vi "Periodic Tasks.vi"(8 "error in":errorcluster) -> ()   [LabVIEW 2023]
doc: "This VI runs in parallel to other tasks. It can contain as many user-defined periodic loops as you need. These can carry out PID or other sorts of timed response."
uses:
  <vilib>/Rock Robotics/WPI/Utilities/WPI_GetSetVariantRefNum.vi
  Robot Global Data.vi
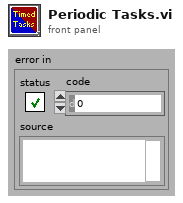
[diagram p1: front panel]
types:
  T1 = typedef "WPI_JoystickDevRef.ctl" = cluster{"Device":T2}
  T2 = typedef "WPI_JoystickDeviceEnum.ctl" = enum16{"USB 0", "USB 1", "USB 2", "USB 3", "USB 4", "USB 5"}
  T3 = typedef "WPI_RobotDriveDevRef.ctl" = cluster{"DevStatus":errorcluster, "Motors[]":T4[], "Square Inputs":bool, "Max Output":dbl}
  T4 = typedef "WPI_MotorControlDeviceRef.ctl" = cluster{"DeviceStatus":errorcluster, "Type":T5, "PWM":cluster{"PWM Channel":T6, "DeadBand":T7}, "CAN":cluster{"Device Number":u8, "SetOutput VI Ref":variant, "GetOutput VI Ref":variant, "Enable VI Ref":variant, "Disable VI Ref":variant, "Data":variant}, "Invert":bool, "DIO PWM":cluster{"PWM \"Enable\" Channel":T6, "DIOChannel":T8, "PWM Rate":dbl}}
  T5 = typedef "WPI_MotorControlType.ctl" = enum16{"PWM", "CAN", "DIO PWM"}
  T6 = typedef "FPGA_DIOPWMChannel.ctl" = enum8{"PWM 0", "PWM 1", "PWM 2", "PWM 3", "PWM 4", "PWM 5", "PWM 6", "PWM 7", "PWM 8", "PWM 9", "PWM MXP 0", "PWM MXP 1", "PWM MXP 2", "PWM MXP 3", "PWM MXP 4", "PWM MXP 5", "PWM MXP 6", "PWM MXP 7", "PWM MXP 8", "PWM MXP 9", "Invalid"}
  T7 = typedef "WPI_PWMDeadband.ctl" = cluster{"Name":string, "maxPositivePwm":i32, "minPositivePwm":i32, "centerPwm":i32, "maxNegativePwm":i32, "minNegativePwm":i32, "angularRange":u16}
  T8 = typedef "FPGA_DIOChannel.ctl" = enum8{"DIO 0", "DIO 1", "DIO 2", "DIO 3", "DIO 4", "DIO 5", "DIO 6", "DIO 7", "DIO 8", "DIO 9", "DIO MXP 0", "DIO MXP 1", "DIO MXP 2", "DIO MXP 3", "DIO MXP 4", "DIO MXP 5", "DIO MXP 6", "DIO MXP 7", "DIO MXP 8", "DIO MXP 9", "DIO MXP 10", "DIO MXP 11", "DIO MXP 12", "DIO MXP 13", "DIO MXP 14", "DIO MXP 15", "SPI Port CS1", "SPI Port CS2", "SPI Port CS3", "SPI Port MISO", "SPI Port MOSI", "Invalid"}
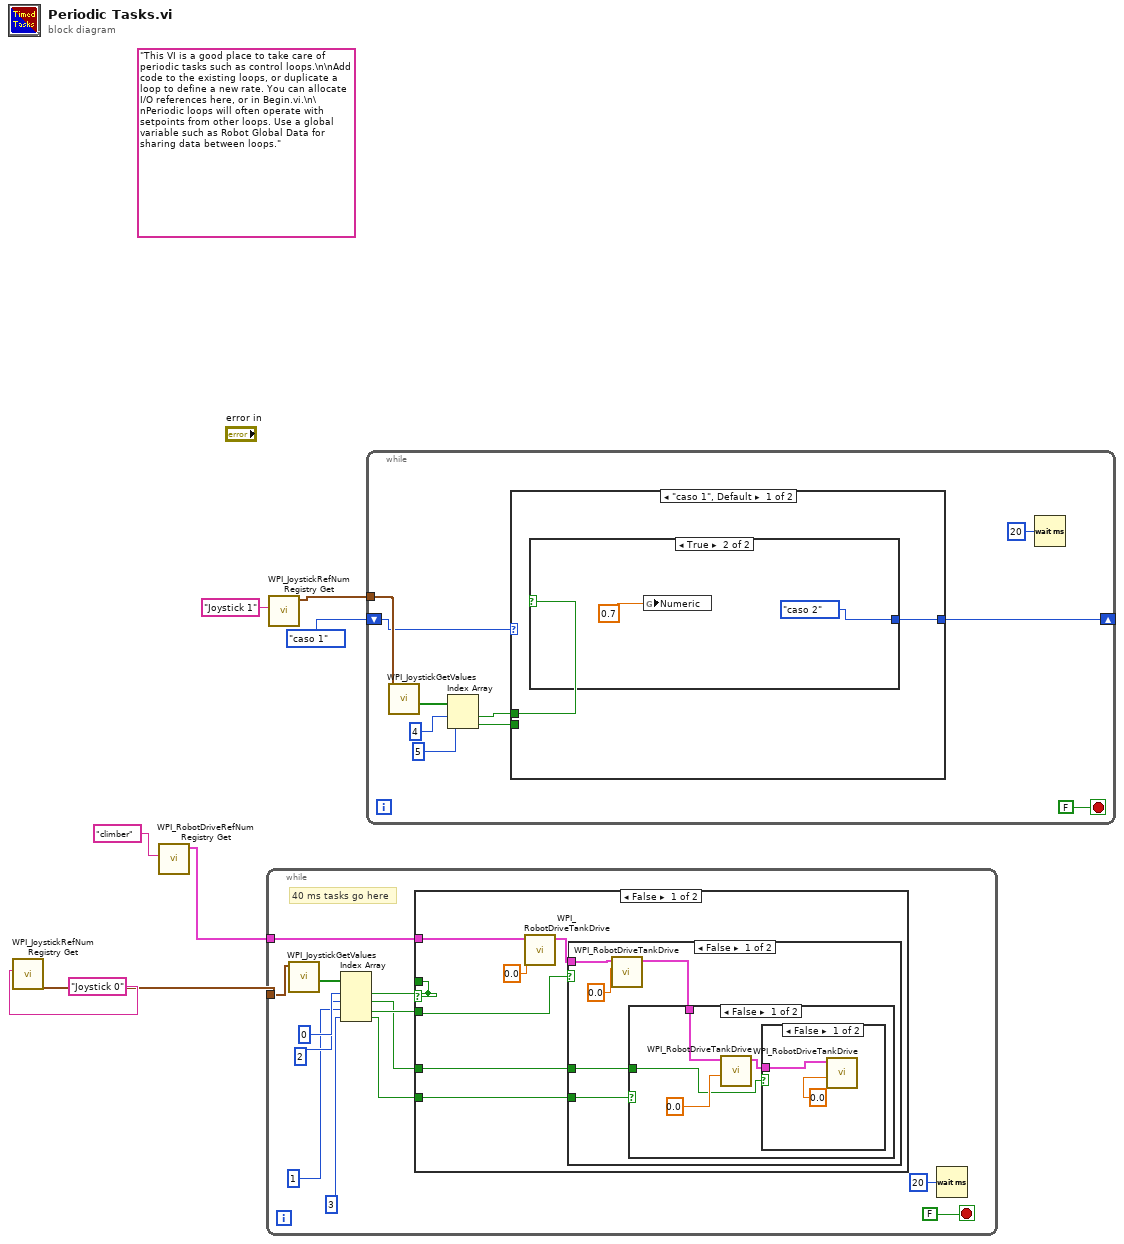
[diagram p0: block diagram]
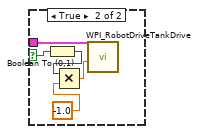
[diagram p2: hidden frame]
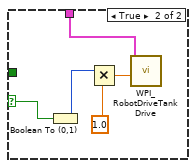
[diagram p3: hidden frame]
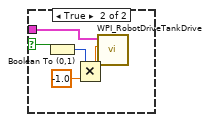
[diagram p4: hidden frame]
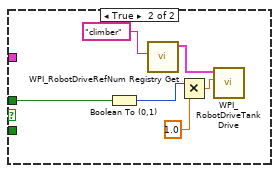
[diagram p5: hidden frame]
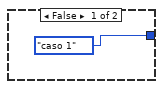
[diagram p6: hidden frame]
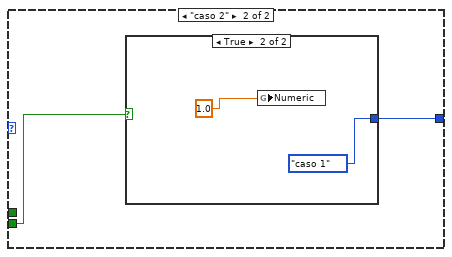
[diagram p7: hidden frame]
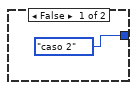
[diagram p8: hidden frame]
diagram:
  (unwired) "This VI is a good place to take care of periodic tasks such as control loops.\n\nAdd code to the existing loops, or duplicate a loop to define a new rate. You can allocate I/O references here, or in Begin.vi.\n\nPeriodic loops will often operate with setpoints from other loops. Use a global variable such as Robot Global Data for sharing data between loops."
  n1 = call <vilib>:"WPI_JoystickRefNum Registry Get.vi"("refnum name"="Joystick 0") -> ("JoystickDevRef"=w3:T1)  [unwired: 1 in, 9 out]
  n2 = call <vilib>:"WPI_RobotDriveRefNum Registry Get.vi"("refnum name"="climber") -> ("RobotDriveDevRef"=w1:T3)  [unwired: 1 in, 9 out]
  n3 = while {
    tunnel: w3 -> [w19]
    tunnel: w1 -> [w10]
    stop <- FALSE stop-if-true
    # "40 ms tasks go here"
    n4 = call <vilib>:"WPI_JoystickGetValues.vi"("JoystickDevRef"=w19) -> ("Buttons"=w17:bool[])  [unwired: 6 in, 4 out]
    n5 = Index Array(array=w17, index #1=0 ("index"), index #2=2 ("index"), index #3=1 ("index"), index #4=3 ("index")) -> (element #1=w11:bool, element #2=w8:bool, element #3=w14:bool, element #4=w9:bool)
    n6 = case shown="False" w11 {
      tunnel: w14 -> [w25 _]
      tunnel: w11 -> [_ w55]
      tunnel: w10 -> [w23 _]
      tunnel: w9 -> [w22 _]
      tunnel: w8 -> [w21 _]
      frame False {
        n7 = call <vilib>:"WPI_RobotDriveTankDrive.vi"("Left axis value"=0.0, "RobotDriveDevRef"=w23) -> ("RobotDriveDevRef"=w24:T3)  [unwired: 7 in, 2 out]
        n8 = case shown="False" w25 {
          selector: w25 -> [_ w51]
          tunnel: w24 -> [w31 w52]
          tunnel: w22 -> [w28 _]
          tunnel: w21 -> [w27 _]
          frame False {
            n9 = call <vilib>:"WPI_RobotDriveTankDrive.vi"("Left axis value"=0.0, "RobotDriveDevRef"=w31) -> ("RobotDriveDevRef"=w29:T3)  [unwired: 7 in, 2 out]
            n10 = case shown="False" w28 {
              selector: w28 -> [_ w47]
              tunnel: w29 -> [w33 w43]
              tunnel: w27 -> [w32 _]
              frame False {
                n11 = call <vilib>:"WPI_RobotDriveTankDrive.vi"("Right axis value"=0.0 ("Left axis value"), "RobotDriveDevRef"=w33) -> ("RobotDriveDevRef"=w34:T3)  [unwired: 7 in, 2 out]
                n12 = case shown="False" w32 {
                  selector: w32 -> [_ w40]
                  tunnel: w34 -> [w37 w42]
                  frame False {
                    n13 = call <vilib>:"WPI_RobotDriveTankDrive.vi"("Right axis value"=0.0 ("Left axis value"), "RobotDriveDevRef"=w37) -> ()  [unwired: 7 in, 3 out]
                  }
                  frame True {
                    n14 = Boolean To (0,1)(Boolean=w40) -> (0, 1=w39:i16)
                    n15 = Multiply(x=w39, y=-1.0) -> (x*y=w38:dbl)
                    n16 = call <vilib>:"WPI_RobotDriveTankDrive.vi"("Right axis value"=w38, "RobotDriveDevRef"=w42) -> ()  [unwired: 7 in, 3 out]
                  }
                }
              }
              frame True {
                n17 = Boolean To (0,1)(Boolean=w47) -> (0, 1=w46:i16)
                n18 = Multiply(x=w46, y=1.0 ("Left axis value")) -> (x*y=w44:dbl)
                n19 = call <vilib>:"WPI_RobotDriveTankDrive.vi"("Right axis value"=w44, "RobotDriveDevRef"=w43) -> ()  [unwired: 7 in, 3 out]
              }
            }
          }
          frame True {
            n20 = Boolean To (0,1)(Boolean=w51) -> (0, 1=w50:i16)
            n21 = Multiply(x=w50, y=-1.0) -> (x*y=w48:dbl)
            n22 = call <vilib>:"WPI_RobotDriveTankDrive.vi"("Left axis value"=w48, "RobotDriveDevRef"=w52) -> ()  [unwired: 7 in, 3 out]
          }
        }
      }
      frame True {
        n23 = Boolean To (0,1)(Boolean=w55) -> (0, 1=w58:i16)
        n24 = call <vilib>:"WPI_RobotDriveRefNum Registry Get.vi"("refnum name"="climber") -> ("RobotDriveDevRef"=w54:T3)  [unwired: 1 in, 9 out]
        n25 = Multiply(x=w58, y=1.0 ("Left axis value")) -> (x*y=w56:dbl)
        n26 = call <vilib>:"WPI_RobotDriveTankDrive.vi"("Left axis value"=w56, "RobotDriveDevRef"=w54) -> ()  [unwired: 7 in, 3 out]
      }
    }
    n27 = Wait (ms)(milliseconds to wait=u32 20) -> ()  [unwired: 1 out]
  }
  n28 = call <vilib>:"WPI_JoystickRefNum Registry Get.vi"("refnum name"="Joystick 1") -> ("JoystickDevRef"=w6:T1)  [unwired: 9 in, 1 out]
  n29 = while {
    tunnel: w6 -> [w67]
    shift-right: [w60] -> _
    shift-left: enum16{"caso 1", "caso 2"}."caso 1" -> [w63]
    stop <- FALSE stop-if-true
    n30 = call <vilib>:"WPI_JoystickGetValues.vi"("JoystickDevRef"=w67) -> ("Buttons"=w66:bool[])  [unwired: 6 in, 4 out]
    n31 = Index Array(array=w66, index #1=4 ("index"), index #2=5 ("index")) -> (element #1=w62:bool, element #2=w61:bool)
    n32 = case shown="\"caso 1\", Default" w63 {
      tunnel: w62 -> [w70 _]
      tunnel: w61 -> [_ w75]
      tunnel: [w69 w74] -> w60
      frame "caso 1", Default {
        n33 = case shown="True" w70 {
          tunnel: [enum16{"caso 1", "caso 2"}."caso 1" enum16{"caso 1", "caso 2"}."caso 2"] -> w69
          frame False {
          }
          frame True {
            n34 = global write "Robot Global Data.vi" "Numeric"(0.7) -> ()
          }
        }
      }
      frame "caso 2" {
        n35 = case shown="True" w75 {
          tunnel: [enum16{"caso 1", "caso 2"}."caso 2" enum16{"caso 1", "caso 2"}."caso 1"] -> w74
          frame False {
          }
          frame True {
            n36 = global write "Robot Global Data.vi" "Numeric"(1.0) -> ()
          }
        }
      }
    }
    n37 = Wait (ms)(milliseconds to wait=u32 20) -> ()  [unwired: 1 out]
  }
